vi "Create.vi"(5 "Page Segmentation Mode (Default: PSM Auto)":T1=enum."PSM_AUTO", 7 "OCR Enginer Mode (Default: OEM Default)":T2=enum."OEM_DEFAULT", 8 "error in (no error)":errorcluster, 9 "White List (Empty: Use Default)":string, 10 "Language Path (Empty: Use Default)":path, 11 "Data Path (Empty: Use System Path)":path) -> (0 "error out":errorcluster, 3 "Text Tesseract":refnum<class "Text Tesseract.lvclass">)   [LabVIEW 2020, in "feature_detection.lvlib" / "Text Tesseract.lvclass"]
doc: "Create a Tesseract OCR instance.\n\nSee https://github.com/tesseract-ocr/tessdoc/blob/main/Installation.md to understand how to install the necessary dependencies."
uses:
  Text Tesseract.lvclass
  Text Tesseract.lvclass/Text Tesseract.ctl
  common/common.lvlib
  common/bin/gartoolkit_tesseract_32-1.dll
  OCR Engine Mode.ctl
  Page Segmentation Mode.ctl
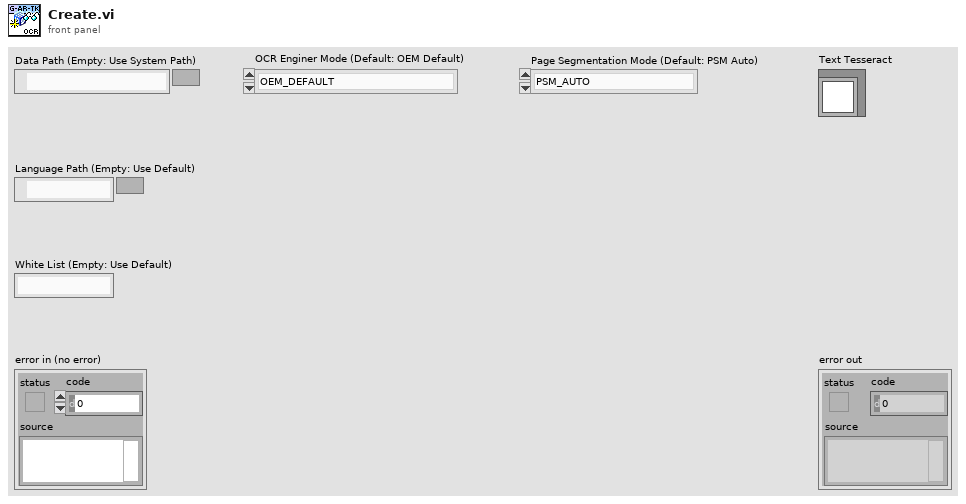
[diagram p1: front panel]
types:
  T1 = typedef "feature_detection.lvlib/Text Tesseract.lvclass/Page Segmentation Mode.ctl" = enum8{"PSM_OSD_ONLY", "PSM_AUTO_OSD", "PSM_AUTO_ONLY", "PSM_AUTO", "PSM_SINGLE_COLUMN", "PSM_SINGLE_BLOCK_VERT_TEXT", "PSM_SINGLE_BLOCK", "PSM_SINGLE_LINE", "PSM_SINGLE_WORD", "PSM_CIRCLE_WORD", "PSM_SINGLE_CHAR"}
  T2 = typedef "feature_detection.lvlib/Text Tesseract.lvclass/OCR Engine Mode.ctl" = enum8{"OEM_TESSERACT_ONLY", "OEM_CUBE_ONLY", "OEM_TESSERACT_CUBE_COMBINED", "OEM_DEFAULT"}
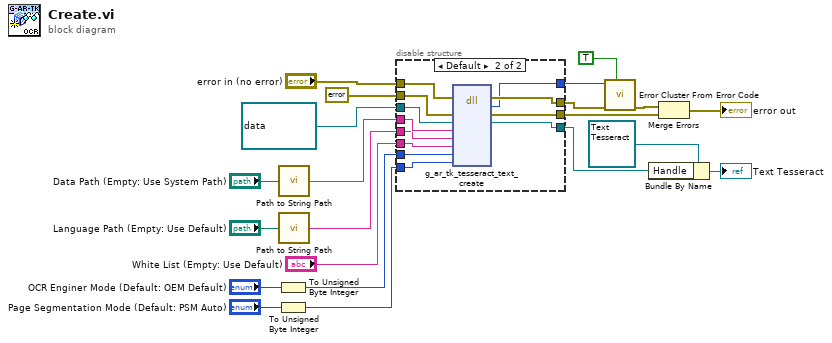
[diagram p0: block diagram]
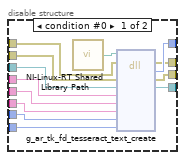
[diagram p2: hidden frame]
diagram:
  n1 = To Unsigned Byte Integer(number="OCR Enginer Mode (Default: OEM Default)") -> (unsigned 8bit integer=w4:u8)
  n2 = To Unsigned Byte Integer(number="Page Segmentation Mode (Default: PSM Auto)") -> (unsigned 8bit integer=w2:u8)
  n3 = call "Path to String Path.vi"("Path"="Data Path (Empty: Use System Path)") -> ("String"=w7:string)
  n4 = call "Path to String Path.vi"("Path"="Language Path (Empty: Use Default)") -> ("String"=w6:string)
  n5 = disable-structure "Conditional Disable Structure" shown="Default" {
    disable-tunnel: "error in (no error)" -> [w32 w46]
    disable-tunnel: errorcluster {"status"=FALSE, "code"=0, "source"=""} ("error constant") -> [w31 w45]
    disable-tunnel: refnum<data-value> refnum ("EDVR") -> [w29 w44]
    disable-tunnel: [w22 w43] -> w18
    disable-tunnel: [w33 w42] -> w17
    disable-tunnel: [w23 w41] -> w16
    disable-tunnel: [w30 w40] -> w15
    disable-tunnel: w7 -> [w28 w39]
    disable-tunnel: w6 -> [w27 w38]
    disable-tunnel: w4 -> [w25 w37]
    disable-tunnel: w2 -> [w24 w36]
    disable-tunnel: "White List (Empty: Use Default)" -> [w26 w35]
    frame condition #0 {
      n6 = call "NI-Linux-RT Shared Library Path.vi"() -> ("Path"=w34:path)
      n7 = dll-call lib="?" fn="g_ar_tk_fd_tesseract_text_create" ("g_ar_toolkit.*.*:g_ar_tk_capture_context_create")(path in=w34, error in=w32, "error_cluster"=w31, "EDVR"=w29, "data_path"=w28, "lang"=w27, "whitelist"=w26, "oem"=w25, "psm"=w24) -> (error out=w22:errorcluster, "return type"=w33:i32, "error_cluster"=w30:errorcluster, "EDVR"=w23:refnum<data-value>)  [unwired: 6 in, 1 out]
    }
    frame condition #1 (active) {
      n8 = dll-call lib="C:/serenial/lib/g-augmented-reality-toolkit/LabVIEW/common/bin/gartoolkit_tesseract_*-1.*" fn="g_ar_tk_tesseract_text_create" ("g_ar_toolkit.*.*:g_ar_tk_capture_context_create")(error in=w46, "error_cluster"=w45, "EDVR"=w44, "data_path"=w39, "lang"=w38, "whitelist"=w35, "oem"=w37, "psm"=w36) -> (error out=w43:errorcluster, "return type"=w42:i32, "error_cluster"=w40:errorcluster, "EDVR"=w41:refnum<data-value>)  [unwired: 7 in, 1 out]
    }
  }
  n9 = call <vilib>:"Error Cluster From Error Code.vi"("show call chain? (False)"=TRUE, "error in (no error)"=w18, "error code (0)"=w17) -> ("error out"=w21:errorcluster)  [unwired: 6 in]
  n10 = Bundle By Name(cluster=refnum<class "Text Tesseract.lvclass"> refnum ("Text Detector in"), "Handle"=w16) -> (→"Text Tesseract":refnum<class "Text Tesseract.lvclass">)
  n11 = Merge Errors(w21, w15) -> (→"error out":errorcluster)
